vi "ErrorMSG_Error_queue.vi"(7 "Method":enum16{"Initial", "Add", "Read", "Delete"}(ring), 8 "error in (no error)":errorcluster, 10 "dequeue timeout(150)":i32=150, 11 "queue element":errorcluster) -> (0 "error out":errorcluster, 2 "timed out?":bool, 3 "dequeue element":errorcluster)   [LabVIEW 2019]
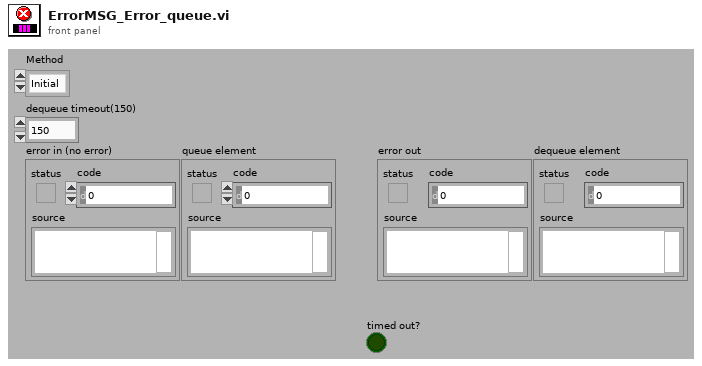
[diagram p1: front panel]
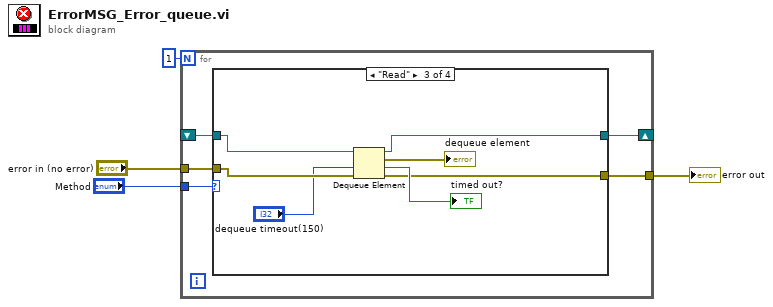
[diagram p0: block diagram]
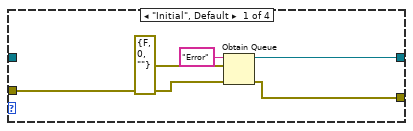
[diagram p2: hidden frame]
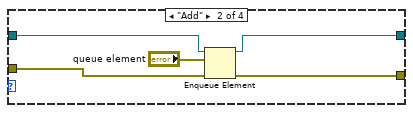
[diagram p3: hidden frame]
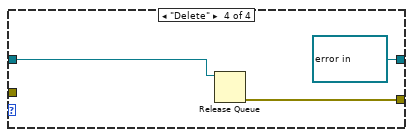
[diagram p4: hidden frame]
diagram:
  n1 = for {
    N: 1 -> [_]
    tunnel: "Method" -> [w9]
    tunnel: [w8] -> w3
    shift-right: [w7] -> _
    shift-left: _ -> [w6]
    tunnel: "error in (no error)" -> [w5]
    n2 = case shown="\"Read\"" w9 {
      tunnel: [w10 w19 w21 w29] -> w8
      tunnel: [w12 w16 w23 refnum<queue> refnum ("queue out")] -> w7
      tunnel: w6 -> [_ w17 w24 w28]
      tunnel: w5 -> [w11 w15 w22 _]
      frame "Initial", Default {
        n3 = Obtain Queue(name (unnamed)="Error", element data type=errorcluster {"status"=FALSE, "code"=0, "source"=""} ("error in"), error in (no error)=w11) -> (queue out=w12:refnum<queue>, error out=w10:errorcluster)  [unwired: 2 in, 1 out]
      }
      frame "Add" {
        n4 = Enqueue Element(queue=w17, element="queue element", error in (no error)=w15) -> (queue out=w16:refnum<queue>, error out=w19:errorcluster)  [unwired: 1 in, 1 out]
      }
      frame "Read" {
        n5 = Dequeue Element(queue=w24, timeout in ms (-1)="dequeue timeout(150)", error in (no error)=w22) -> (queue out=w23:refnum<queue>, element=→"dequeue element":errorcluster, timed out?=→"timed out?":bool, error out=w21:errorcluster)
      }
      frame "Delete" {
        n6 = Release Queue(queue=w28) -> (error out=w29:errorcluster)  [unwired: 2 in, 2 out]
      }
    }
  }
  "error out" <- w3
